vi "Queue FG.vi"(7 "Queue Reference Actions":T1, 8 "error in":errorcluster, 11 "Queue in":refnum<queue>) -> (0 "error out":errorcluster, 3 "Queue out":refnum<queue>)   [LabVIEW 2015, in "Generic Module Library.lvlib" / "Template G_Module.lvlib"]
uses:
  Template G_Module.lvlib
  Private Controls/Module Message Cluster.ctl
  Private Controls/Module Message Cluster Components/Acknowledge Data Cluster.ctl
  Private Controls/Module Message Cluster Components/Message Data Cluster.ctl
  Private Controls/Module Message Cluster Components/Ack Payload.ctl
  Queue Reference Actions.ctl
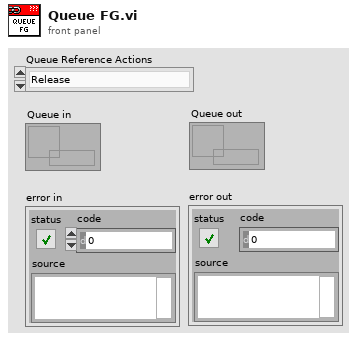
[diagram p1: front panel]
types:
  T1 = typedef "Generic Module Library.lvlib/Template G_Module.lvlib/Queue Reference Actions.ctl" = enum16{"Release", "Set", "Get"}
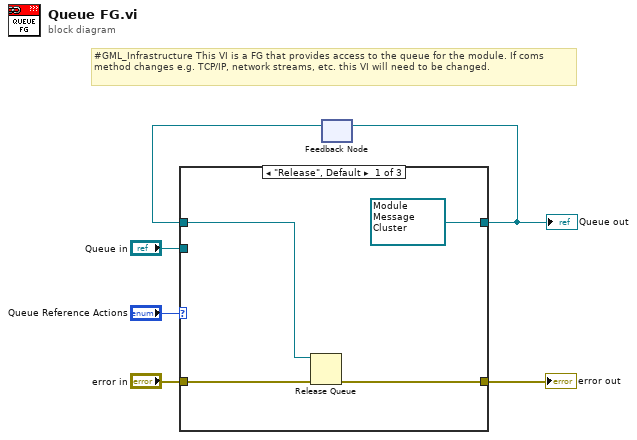
[diagram p0: block diagram]
diagram:
  # "#GML_Infrastructure This VI is a FG that provides access to the queue for the module. If coms method changes e.g. TCP/IP, network streams, etc. this VI will need to be changed."
  n1 = feedback #1() -> (w5:refnum<queue>)  [unwired: 1 in]
  n2 = case shown="\"Release\", Default" "Queue Reference Actions" {
    tunnel: "Queue in" -> [_ _ w13]
    tunnel: w5 -> [w10 w12 _]
    tunnel: [refnum<queue> refnum ("Queue in") w12 w13] -> w1
    tunnel: "error in" -> [w9 w11 w14]
    tunnel: [w8 w11 w14] -> w3
    frame "Release", Default {
      n3 = Release Queue(queue=w10, error in (no error)=w9) -> (error out=w8:errorcluster)  [unwired: 1 in, 2 out]
    }
    frame "Get" {
    }
    frame "Set" {
    }
  }
  "Queue out" <- w1
  "error out" <- w3
  n4 = feedback-in #1(w1) -> ()
